vi "CleanUp.vi"(0 "object in":refnum<class "NISwitch.lvclass">, 5 "error in (no error)":errorcluster) -> (14 "object out":refnum<class "NISwitch.lvclass">, 19 "error out":errorcluster)   [LabVIEW 2023, in "HardwareAbstractionLayer_LVOOP.lvlib" / "NISwitch.lvclass"]
uses:
  NISwitch.lvclass
  NISwitch.lvclass/NISwitch.ctl
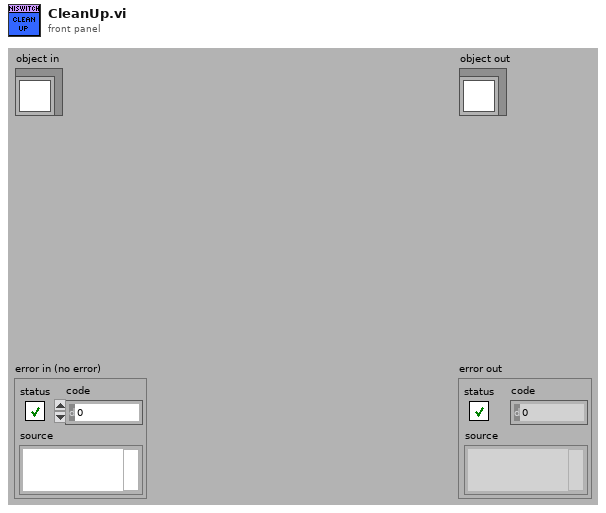
[diagram p1: front panel]
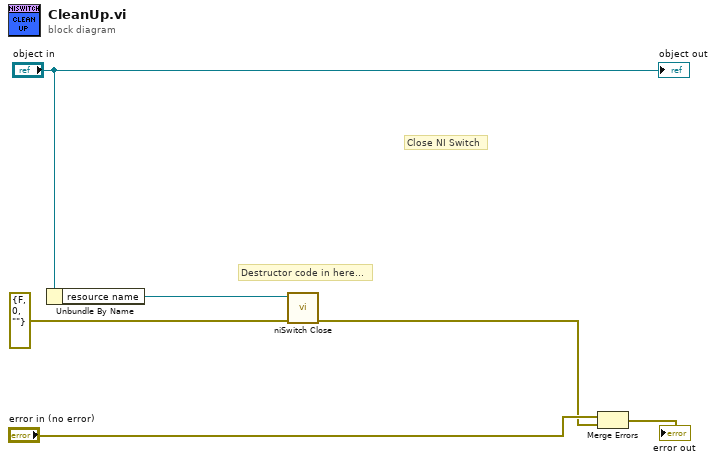
[diagram p0: block diagram]
diagram:
  # "Close NI Switch"
  # "Destructor code in here..."
  n1 = Unbundle By Name("object in") -> ("resource name"=w1:refnum<k15>)
  n2 = call <instrlib>:"niSwitch Close.vi"("error in (no error)"=errorcluster {"status"=FALSE, "code"=0, "source"=""}, "instrument handle"=w1) -> ("error out"=w2:errorcluster)  [unwired: 9 in]
  n3 = Merge Errors("error in (no error)", w2) -> (→"error out":errorcluster)
  "object out" <- "object in"
